vi "Auto Configure DAQ.vi"(8 "error in (no error)":errorcluster, 11 "Instrument.DAQ":refnum<class "Instrument.DAQ.lvclass">) -> (0 "error out":errorcluster, 3 "Instrument.DAQ out":refnum<class "Instrument.DAQ.lvclass">)   [LabVIEW 2019, in "Instrument.Lockin.lvlib" / "Instrument.DAQ.lvclass"]
uses:
  Instrument.DAQ.lvclass
  <resource>/objmgr/daqmx.rc
  Typedefs/DAQ.Config.AI.Range--enum.ctl
  Typedefs/DAQ.Config.AI.Coupling--enum.ctl
  Typedefs/DAQ.Config.AO.Range--enum.ctl
  Typedefs/DAQ.Type--enum.ctl
  Typedefs/DAQ.Config.AI--Cluster.ctl
  Typedefs/DAQ.Config.AO--Cluster.ctl
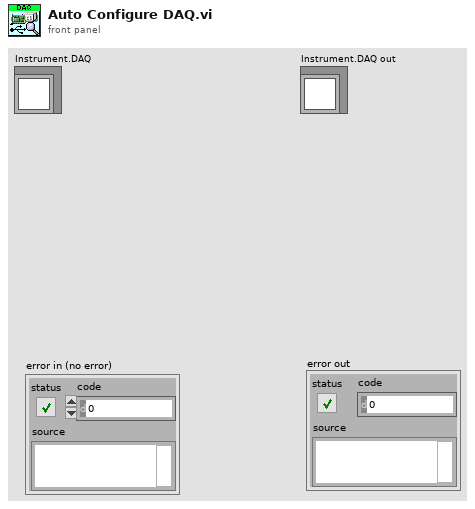
[diagram p1: front panel]
types:
  T1 = typedef "Instrument.Lockin.lvlib/Instrument.DAQ.lvclass/DAQ.Config.AI--Cluster.ctl" = cluster{"Channels":tag, "Coupling":T2, "Range":T3, "input terminal configuration":i32, "Type":T4}
  T2 = typedef "Instrument.Lockin.lvlib/Instrument.DAQ.lvclass/DAQ.Config.AI.Coupling--enum.ctl" = u16
  T3 = typedef "Instrument.Lockin.lvlib/Instrument.DAQ.lvclass/DAQ.Config.AI.Range--enum.ctl" = enum16{"±0.316", "±1.00", "±3.16", "±10.0", "±31.6", "±42.4"}
  T4 = typedef "Instrument.Lockin.lvlib/Instrument.DAQ.lvclass/DAQ.Type--enum.ctl" = enum16{"None", "USB-4431", "PXI-446x"}
  T5 = typedef "Instrument.Lockin.lvlib/Instrument.DAQ.lvclass/DAQ.Config.AO--Cluster.ctl" = cluster{"Channels":tag, "Range":T6, "output terminal configuration":i32, "Type":T4}
  T6 = typedef "Instrument.Lockin.lvlib/Instrument.DAQ.lvclass/DAQ.Config.AO.Range--enum.ctl" = enum16{"±0.1", "±1.0", "±10.0"}
  T7 = typedef "Instrument.Lockin.lvlib/Instrument.DAQ.lvclass/DeviceInfo--Cluster.ctl" = cluster{"DeviceName":string, "DevIsSimulated":bool, "DeviceSerialNumber":u32, "ProductType":string, "ProductCategory":i32, "ProductNumber":u32, "ChassisNumber":u32, "SlotNumber":u32, "ChassisName":string, "ChassisSerialNumber":string}
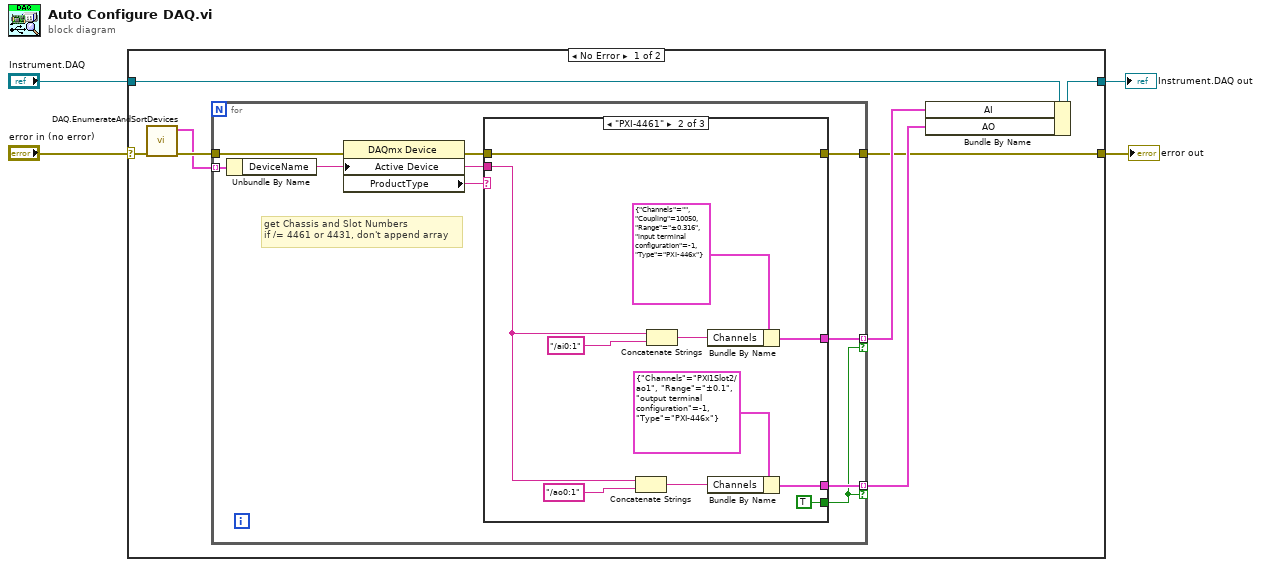
[diagram p0: block diagram]
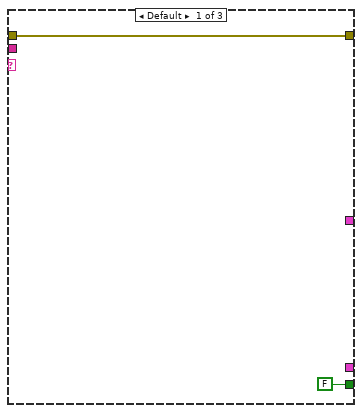
[diagram p2: hidden frame]
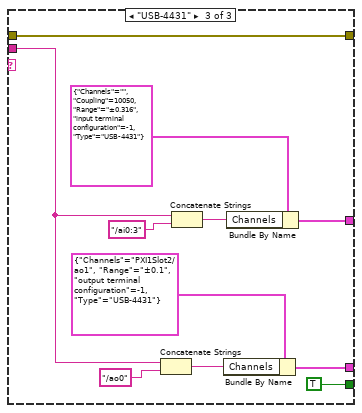
[diagram p3: hidden frame]
diagram:
  n1 = case shown="No Error" "error in (no error)" {
    selector: "error in (no error)" -> [w9 w46]
    tunnel: [w10 w46] -> w4
    tunnel: "Instrument.DAQ" -> [w7 w47]
    tunnel: [w6 w47] -> w2
    frame No Error {
      n2 = call "DAQ.EnumerateAndSortDevices.vi"("error in (no error)"=w9) -> ("error out"=w8:errorcluster, "Devices (sorted)"=w5:T7[])  [unwired: 9 in]
      n3 = for {
        tunnel: [w16] -> w10
        tunnel: [w21] -> w12 mode=indexing if=w18
        tunnel: [w20] -> w11 mode=indexing if=w18
        tunnel: w8 -> [w15]
        tunnel: w5 -> [w14] mode=indexing
        # "get Chassis and Slot Numbers\nif /= 4461 or 4431, don't append array"
        n4 = Unbundle By Name(w14) -> ("DeviceName"=w13:string)
        n5 = property class="DAQmx Device"(error in=w15, "Active Device"=w13) -> (error out=w17:errorcluster, "ProductType"=w19:string)  [unwired: 1 in, 1 out]
        n6 = case shown="\"PXI-4461\"" w19 {
          tunnel: [_ w30 w41] -> w21
          tunnel: [_ w29 w40] -> w20
          tunnel: [FALSE TRUE TRUE] -> w18
          tunnel: w17 -> [w22 w25 w35]
          tunnel: [w22 w25 w35] -> w16
          tunnel: w13 -> [_ w24 w36]
          frame Default {
          }
          frame "PXI-4461" {
            n7 = Concatenate Strings(w24, "/ao0:1" ("string")) -> (w33:string)
            n8 = Concatenate Strings(w24, "/ai0:1" ("string")) -> (w27:string)
            n9 = Bundle By Name(cluster=T1 {"Channels"="", "Coupling"=10050, "Range"=enum."±0.316", "input terminal configuration"=-1, "Type"=enum."PXI-446x"} ("AI.Config"), "Channels"=w27) -> (w30:T1)
            n10 = Bundle By Name(cluster=T5 {"Channels"="PXI1Slot2/ao1", "Range"=enum."±0.1", "output terminal configuration"=-1, "Type"=enum."PXI-446x"} ("AO.config"), "Channels"=w33) -> (w29:T5)
          }
          frame "USB-4431" {
            n11 = Concatenate Strings(w36, "/ao0" ("string")) -> (w44:string)
            n12 = Concatenate Strings(w36, "/ai0:3" ("string")) -> (w38:string)
            n13 = Bundle By Name(cluster=T5 {"Channels"="PXI1Slot2/ao1", "Range"=enum."±0.1", "output terminal configuration"=-1, "Type"=enum."USB-4431"} ("AO.config"), "Channels"=w44) -> (w40:T5)
            n14 = Bundle By Name(cluster=T1 {"Channels"="", "Coupling"=10050, "Range"=enum."±0.316", "input terminal configuration"=-1, "Type"=enum."USB-4431"} ("AI.Config"), "Channels"=w38) -> (w41:T1)
          }
        }
      }
      n15 = Bundle By Name(cluster=w7, "AI"=w12, "AO"=w11) -> (w6:refnum<class "Instrument.DAQ.lvclass">)
    }
    frame Error {
    }
  }
  "error out" <- w4
  "Instrument.DAQ out" <- w2
